vi "בדיקת זמן מיתוג הממסר 7.vi"(8 "error":errorcluster, 11 "Path for Log":path) -> (0 "error out":errorcluster, 1 "בטוח כן/לא":bool, 2 "בדיקת זמן מיתוג הממסר":dbl, 7 "Userresult":bool)   [LabVIEW 2014]
uses:
  <instrlib>/niDMM/nidmm.llb/niDMM Function.ctl
  <instrlib>/niDMM/nidmm.llb/niDMM Resolution in Digits.ctl
  <vilib>/DAQmx/create/channels.llb/DAQmx Create Channel (DO-Digital Output).vi
  <instrlib>/niDMM/nidmm.llb/niDMM Configure Measurement Digits.vi
  <vilib>/DAQmx/write.llb/DAQmx Write (Digital Bool 1Line 1Point).vi
panel:
  in  "התחל":bool
  # "Right-Click to\nexplain error"
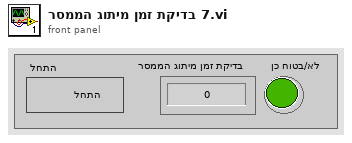
[diagram p1: front panel]
types:
  T1 = enum32{"Invalid", "Standard", "Closed", "Hidden", "Minimized", "Maximized"}
  T2 = typedef "niDMM Function.ctl" = enum16{"DC Volts", "AC Volts", "DC Current", "AC Current", "2-wire Resistance", "4-wire Resistance", "Diode", "Frequency", "Period", "AC Volts DC Coupled", "Capacitance", "Inductance", "Temperature"}
  T3 = typedef "niDMM Resolution in Digits.ctl" = dbl
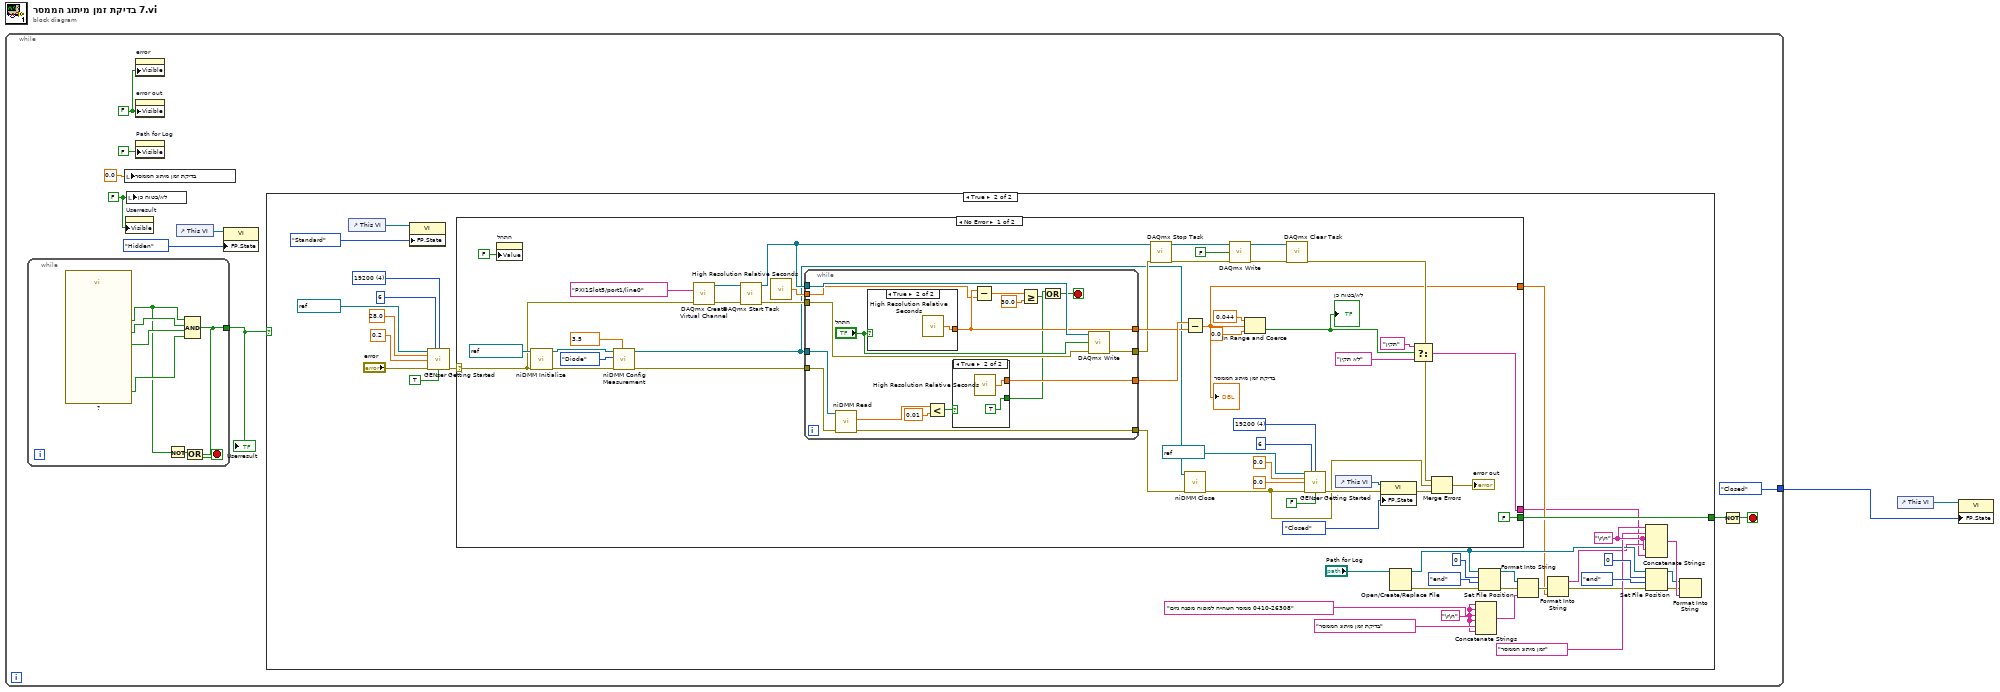
[diagram p0: block diagram]
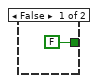
[diagram p2: hidden frame]
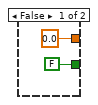
[diagram p3: hidden frame]
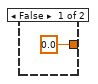
[diagram p4: hidden frame]
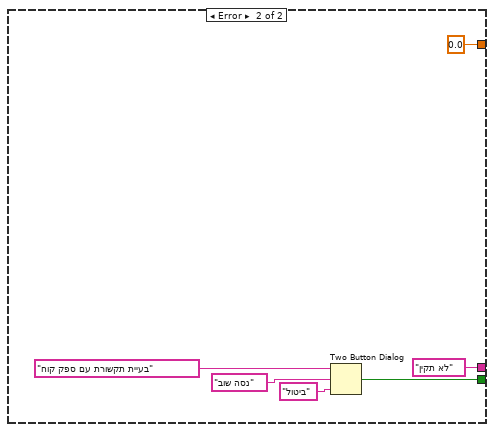
[diagram p5: hidden frame]
diagram:
  n1 = while {
    tunnel: [T1."Closed" ("Front Panel Window:State")] -> w1
    stop <- w10 stop-if-true
    w4 = FALSE ("בטוח כן/לא")
    w11 = FALSE ("Visible")
    n2 = while {
      tunnel: [w13] -> w7
      stop <- w16 stop-if-true
      n3 = call "?"() -> ("הדקי הרב מודד"=w17:bool, "(מגע שלילי (מעטפת"=w18:bool, "C מגע חיובי"=w19:bool, "OK"=w14:bool)  [unwired: 15 in, 1 out]
      n4 = Not(x=w14) -> (.not. x?=w15:bool)
      n5 = Compound Arithmetic op=AND(w14, w19, w18, w17) -> (w13:bool)
      n6 = Or(x=w15, y=w13) -> (x .or. y?=w16:bool)
    }
    "Userresult" <- w7
    n7 = local write "בדיקת זמן מיתוג הממסר"(0.0 ("בדיקת זמן מיתוג הממסר")) -> ()
    n8 = property on="Userresult" class="Bool (strict)"("Visible"=w4) -> ()  [unwired: 2 in, 2 out]
    n9 = local write "בטוח כן/לא"(w4) -> ()
    n10 = property on="error" class="Clust (strict)"("Visible"=w11) -> ()  [unwired: 2 in, 2 out]
    n11 = property on="error out" class="Clust (strict)"("Visible"=w11) -> ()  [unwired: 2 in, 2 out]
    n12 = property on="Path for Log" class="Path"("Visible"=FALSE) -> ()  [unwired: 2 in, 2 out]
    n13 = control-ref of="This VI"() -> (w9:refnum<vi>)
    n14 = property class="VI"(reference=w9, "FP.State"=T1."Hidden" ("Front Panel Window:State")) -> ()  [unwired: 1 in, 2 out]
    n15 = case shown="True" w7 {
      tunnel: [FALSE ("T button?") w47] -> w12
      frame False {
      }
      frame True {
        w31 = "\r\n"
        w38 = "\r\n"
        w50 = u16 4 items=["1200", "2400", "4800", "9600", "19200"] ("BAUD")
        n16 = control-ref of="This VI"() -> (w46:refnum<vi>)
        n17 = property class="VI"(reference=w46, "FP.State"=T1."Standard" ("Front Panel Window:State")) -> ()  [unwired: 1 in, 2 out]
        n18 = call "GENser Getting Started.vi"("VISA"=refnum<visa-resource-name> "COM6", "GEN Addr"=i16 6, "BAUD"=w50, "Voltage Limit"=28.0, "Current Limit"=0.2, "error"="error", "Output On (T)"=TRUE) -> ("error out"=w52:errorcluster)  [unwired: 5 in, 3 out]
        n19 = case shown="No Error" w52 {
          selector: w52 -> [w56 _]
          tunnel: [FALSE ("T button?") w126] -> w47
          tunnel: [w74 0.0] -> w23
          tunnel: [w70 "לא תקין"] -> w22
          frame No Error {
            w62 = T3 3.5 items=["3 1/2"=3.5, "4 1/2"=4.5, "5 1/2"=5.5, "6 1/2"=6.5, "7 1/2"=7.5] ("Resolution in Digits")
            w93 = u16 4 items=["1200", "2400", "4800", "9600", "19200"] ("BAUD")
            n20 = property on="התחל" class="Bool (strict)"("Value"=FALSE ("data")) -> ()  [unwired: 2 in, 2 out]
            n21 = call <instrlib>:"niDMM Initialize.vi"("error in (no error)"=w56, "Instrument Descriptor"=refnum<k15> "PXI1Slot9") -> ("error out"=w60:errorcluster, "instrument handle out"=w61:refnum<k15>)  [unwired: 8 in]
            n22 = call-poly <instrlib>:"niDMM Config Measurement.vi"("Resolution in Digits"=w62, "error in (no error)"=w60, "Function"=niDMM_Function."Diode", "instrument handle"=w61) -> ("error out"=w59:errorcluster, "instrument handle out"=w57:refnum<k15>)  [unwired: 6 in]
            n23 = call-poly <vilib>:"DAQmx Create Virtual Channel.vi"("lines"=tag "PXI1Slot5/port1/line0", "error in"=w56) -> ("task out"=w67:refnum<k21>, "error out"=w68:errorcluster)  [unwired: 12 in]
            n24 = call <vilib>:"DAQmx Start Task.vi"("task/channels in"=w67, "error in"=w68) -> ("task out"=w58:refnum<k21>, "error out"=w65:errorcluster)  [unwired: 12 in]
            n25 = call <vilib>:"High Resolution Relative Seconds.vi"() -> ("relative seconds"=w64:dbl)
            n26 = while {
              tunnel: [w109] -> w82
              tunnel: [w117] -> w83
              tunnel: [w116] -> w81
              tunnel: [w111] -> w80
              tunnel: w58 -> [w115]
              tunnel: w65 -> [w114]
              tunnel: w64 -> [w108]
              tunnel: w59 -> [w101]
              tunnel: w57 -> [w100]
              stop <- w105 stop-if-true
              n27 = call <instrlib>:"niDMM Read.vi"("error in (no error)"=w101, "instrument handle"=w100) -> ("error out"=w111:errorcluster, "Measurement"=w113:dbl)  [unwired: 7 in, 1 out]
              n28 = case shown="True" "התחל" {
                tunnel: [0.0 ("relative seconds") w123] -> w109
                frame False {
                }
                frame True {
                  n29 = call <vilib>:"High Resolution Relative Seconds.vi"() -> ("relative seconds"=w123:dbl)
                }
              }
              n30 = Less?(x=w113, y=0.01) -> (x < y?=w102:bool)
              n31 = case shown="True" w102 {
                tunnel: [0.0 ("relative seconds") w121] -> w117
                tunnel: [FALSE TRUE] -> w104
                frame False {
                }
                frame True {
                  n32 = call <vilib>:"High Resolution Relative Seconds.vi"() -> ("relative seconds"=w121:dbl)
                }
              }
              n33 = Subtract(x=w109, y=w108) -> (x-y=w107:dbl)
              n34 = Greater Or Equal?(x=w107, y=30.0) -> (x >= y?=w103:bool)
              n35 = Or(x=w104, y=w103) -> (x .or. y?=w105:bool)
              n36 = call-poly <vilib>:"DAQmx Write.vi"("task/channels in"=w115, "data"="התחל", "error in"=w114) -> ("error out"=w116:errorcluster)  [unwired: 10 in, 2 out]
            }
            n37 = call <vilib>:"DAQmx Stop Task.vi"("task/channels in"=w58, "error in"=w81) -> ("task out"=w88:refnum<k21>, "error out"=w87:errorcluster)  [unwired: 12 in]
            n38 = Subtract(x=w83, y=w82) -> (x-y=w74:dbl)
            "בדיקת זמן מיתוג הממסר" <- w74
            n39 = call <instrlib>:"niDMM Close.vi"("error in (no error)"=w80, "instrument handle"=w57) -> ("error out"=w55:errorcluster)  [unwired: 9 in]
            n40 = call-poly <vilib>:"DAQmx Write.vi"("task/channels in"=w88, "data"=FALSE, "error in"=w87) -> ("task out"=w85:refnum<k21>, "error out"=w86:errorcluster)  [unwired: 10 in, 1 out]
            n41 = In Range and Coerce(upper limit=0.044, x=w74, lower limit=0.0) -> (In Range?=w71:bool)  [unwired: 1 out]
            "בטוח כן/לא" <- w71
            n42 = call <vilib>:"DAQmx Clear Task.vi"("task in"=w85, "error in"=w86) -> ("error out"=w78:errorcluster)  [unwired: 13 in]
            n43 = call "GENser Getting Started.vi"("VISA"=refnum<visa-resource-name> "COM6", "GEN Addr"=i16 6, "BAUD"=w93, "Voltage Limit"=0.0, "Current Limit"=0.0, "error"=w55, "Output On (T)"=FALSE) -> ("error out"=w92:errorcluster)  [unwired: 5 in, 3 out]
            n44 = control-ref of="This VI"() -> (w91:refnum<vi>)
            n45 = property class="VI"(reference=w91, error in=w92, "FP.State"=T1."Closed" ("Front Panel Window:State")) -> (error out=w77:errorcluster)  [unwired: 1 out]
            n46 = Select(t="תקין", s=w71, f="לא תקין") -> (s? t:f=w70:string)
            n47 = Merge Errors(w78, w55, w77) -> (→"error out":errorcluster)
          }
          frame Error {
            n48 = Two Button Dialog(message="בעיית תקשורת עם ספק קוח", 1:"ביטול" ("F button name (\"Cancel\")"), 2:"נסה שוב" ("T button name (\"OK\")")) -> (T button?=w126:bool)
          }
        }
        n49 = Open/Create/Replace File(file path (use dialog)="Path for Log") -> (refnum out=w27:refnum<file>, error out=w28:errorcluster)  [unwired: 5 in, 1 out]
        n50 = Concatenate Strings(w38, w38, "ממסר השהייה למפוח מפנה גזים 0410-26308", w38, "בדיקת זמן מיתוג הממסר", w38) -> (w41:string)
        n51 = Set File Position(offset (in bytes) (0)=i64 0, refnum=w27, from (0:start)=enum16{"start", "end", "current"}."end", error in=w28) -> (refnum out=w39:refnum<file>, error out=w37:errorcluster)
        n52 = Format Into String(initial string=w39, error in=w37, w41) -> (error out=w26:errorcluster)  [unwired: 1 in, 1 out]
        n53 = Format Into String(error in=w26, w23) -> (resulting string=w24:string, error out=w25:errorcluster)  [unwired: 2 in]
        n54 = Concatenate Strings(w31, "זמן מיתוג הממסר", w31, w24, w31, w22) -> (w36:string)
        n55 = Set File Position(offset (in bytes) (0)=i64 0, refnum=w27, from (0:start)=enum16{"start", "end", "current"}."end", error in=w25) -> (refnum out=w34:refnum<file>, error out=w35:errorcluster)
        n56 = Format Into String(initial string=w34, error in=w35, w36) -> ()  [unwired: 1 in, 2 out]
      }
    }
    n57 = Not(x=w12) -> (.not. x?=w10:bool)
  }
  n58 = control-ref of="This VI"() -> (w2:refnum<vi>)
  n59 = property class="VI"(reference=w2, "FP.State"=w1) -> ()  [unwired: 1 in, 2 out]
